vi "setVipBuildNumber.vi"() -> ()   [LabVIEW 2015]
uses:
  <vilib>/JKI/VIPM API/command-line/support/VI Package Build Spec Data Cluster_vipm_api.ctl
  <vilib>/JKI/VIPM API/command-line/support/Version Info Cluster_vipm_api.ctl
  <vilib>/Utility/error.llb/DialogType.ctl
  <vilib>/JKI/VIPM API/VIPM API_vipm_api.lvlib
  <vilib>/Wiresmith Technology/G CLI/CLI Class/CLI.lvclass
panel:
  out "Next build number":u32
  out "error out":errorcluster
  out "VI Package Build Spec Data":T1
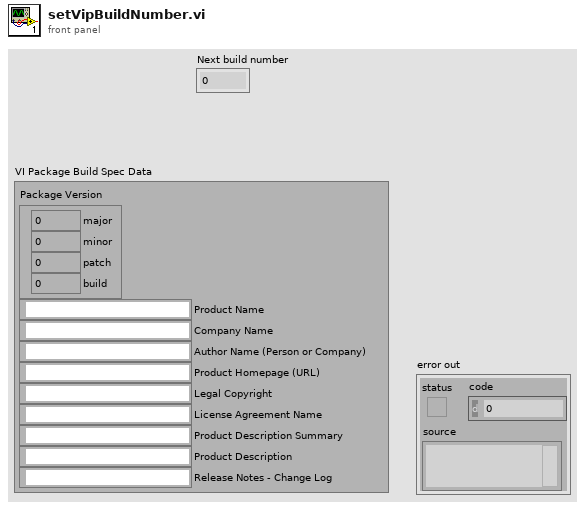
[diagram p1: front panel]
types:
  T1 = typedef "VIPM API_vipm_api.lvlib/VI Package Build Spec Data Cluster_vipm_api.ctl" = cluster{"Package Version":T2, "Product Name":string, "Company Name":string, "Author Name (Person or Company)":string, "Product Homepage (URL)":string, "Legal Copyright":string, "License Agreement Name":string, "Product Description Summary":string, "Product Description":string, "Release Notes - Change Log":string}
  T2 = typedef "VIPM API_vipm_api.lvlib/Version Info Cluster_vipm_api.ctl" = cluster{"major":u32, "minor":u32, "patch":u32, "build":u32}
  T3 = typedef "VIPM API_vipm_api.lvlib/Repository Contents Cluster_vipm_api.ctl" = cluster{"Package Name":string, "Version":string, "Display Name":string, "Release Date":string, "Deprecated":bool}
  T4 = typedef "DialogType.ctl" = u16
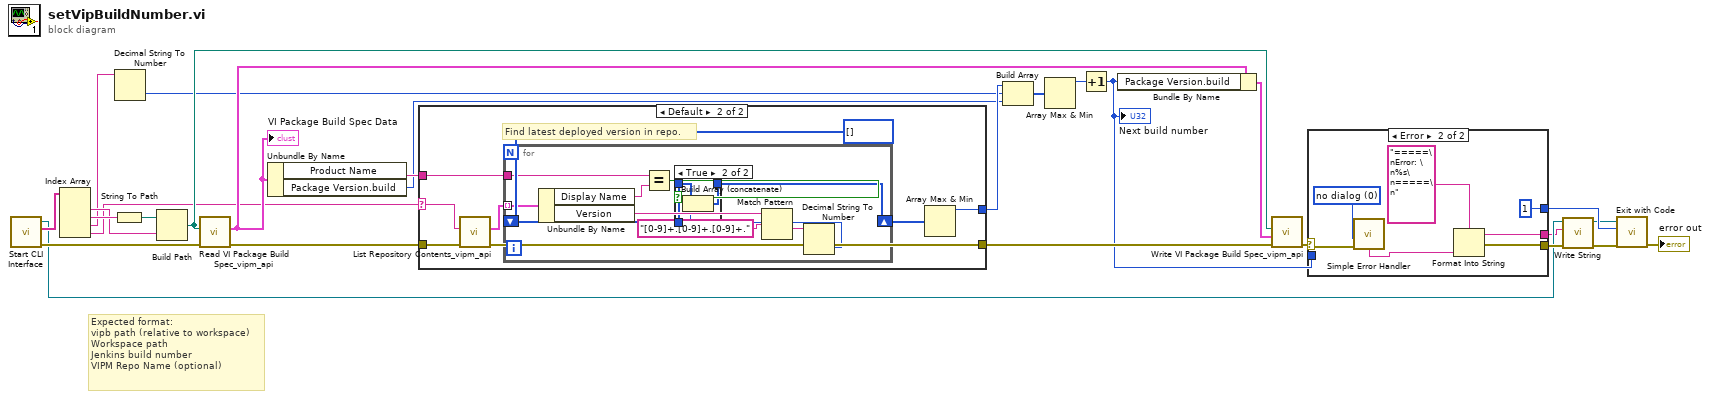
[diagram p0: block diagram]
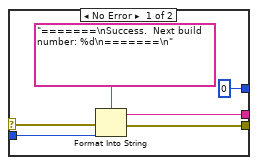
[diagram p2: hidden frame]
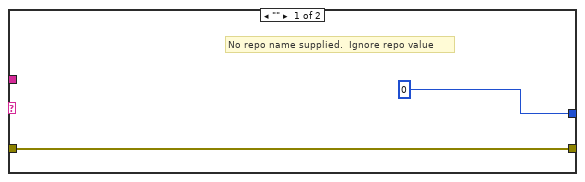
[diagram p3: hidden frame]
diagram:
  # "Expected format:\nvipb path (relative to workspace)\nWorkspace path\nJenkins build number\nVIPM Repo Name (optional)"
  n1 = call <vilib>:"Start CLI Interface.vi"() -> ("error out"=w18:errorcluster, "Custom Parameters"=w16:string[], "CLI out"=w3:refnum<class "CLI.lvclass">)  [unwired: 8 in, 1 out]
  n2 = Index Array(array=w16) -> (element #1=w13:string, element #2=w15:string, element #3=w12:string, element #4=w10:string)  [unwired: 4 in]
  n3 = String To Path(string=w15) -> (path=w14:path)
  n4 = Decimal String To Number(string=w12) -> (number=w11:i32)  [unwired: 2 in, 1 out]
  n5 = Build Path(base path=w14, name or relative path=w13) -> (appended path=w17:path)
  n6 = call <vilib>:"Read VI Package Build Spec_vipm_api.vi"("error in (no error)"=w18, "Path to VIPB File"=w17) -> ("error out"=w23:errorcluster, "VI Package Build Spec Data"=w22:T1)  [unwired: 8 in]
  "VI Package Build Spec Data" <- w22
  n7 = Unbundle By Name(w22) -> ("Product Name"=w21:string, "Package Version.build"=w20:u32)
  n8 = case shown="Default" w10 {
    selector: w10 -> [_ w33]
    tunnel: [0 w31] -> w27
    tunnel: [w28 w36] -> w7
    tunnel: w23 -> [w28 w35]
    tunnel: w21 -> [_ w34]
    frame "" {
      # "No repo name supplied.  Ignore repo value"
    }
    frame Default {
      # "Find latest deployed version in repo."
      n9 = call <vilib>:"List Repository Contents_vipm_api.vi"("error in (no error)"=w35, "Repository Name"=w33) -> ("error out"=w36:errorcluster, "Repository Contents []"=w37:T3[])  [unwired: 7 in, 1 out]
      n10 = for {
        tunnel: w37 -> [w47] mode=indexing
        tunnel: w34 -> [w45]
        shift-right: [w38] -> w32
        shift-left: i32[] [] ("Array") -> [w39]
        n11 = Unbundle By Name(w47) -> ("Display Name"=w46:string, "Version"=w42:string)
        n12 = Equal?(x=w45, y=w46) -> (x = y?=w40:bool)
        n13 = Match Pattern(string=w42, regular expression="[0-9]+.[0-9]+.[0-9]+.") -> (after substring=w43:string)  [unwired: 1 in, 3 out]
        n14 = Decimal String To Number(string=w43) -> (number=w41:i32)  [unwired: 2 in, 1 out]
        n15 = case shown="True" w40 {
          tunnel: w39 -> [w48 w50]
          tunnel: w41 -> [_ w49]
          tunnel: [w48 w51] -> w38
          frame False {
          }
          frame True {
            n16 = Build Array (concatenate)(w50, w49) -> (w51:i32[])
          }
        }
      }
      n17 = Array Max & Min(array=w32) -> (max value=w31:i32)  [unwired: 3 out]
    }
  }
  n18 = Build Array(w27, w11, w20) -> (w26:u32[])
  n19 = Array Max & Min(array=w26) -> (max value=w25:u32)  [unwired: 3 out]
  n20 = Increment(x=w25) -> (x+1=w6:u32)
  "Next build number" <- w6
  n21 = Bundle By Name(cluster=w22, "Package Version.build"=w6) -> (w24:T1)
  n22 = call <vilib>:"Write VI Package Build Spec_vipm_api.vi"("error in (no error)"=w7, "VI Package Build Spec Data"=w24, "Path to VIPB File"=w17) -> ("error out"=w9:errorcluster)  [unwired: 8 in]
  n23 = case shown="Error" w9 {
    selector: w9 -> [w55 w61]
    tunnel: [0 ("Exit Code (0)") 1 ("Exit Code (0)")] -> w8
    tunnel: w6 -> [w54 _]
    tunnel: [w53 w63] -> w4
    tunnel: [w52 w62] -> w2
    frame No Error {
      n24 = Format Into String(format string="=======\nSuccess.  Next build number: %d\n=======\n", error in=w55, w54) -> (resulting string=w52:string, error out=w53:errorcluster)  [unwired: 1 in]
    }
    frame Error {
      w58 = T4 0 items=["no dialog", "OK message", "continue or stop message", "OK message + warnings", "continue/stop + warnings"] ("type of dialog (OK msg:1)")
      n25 = call <vilib>:"Simple Error Handler.vi"("type of dialog (OK msg:1)"=w58, "error in (no error)"=w61) -> ("message"=w59:string)  [unwired: 3 in, 4 out]
      n26 = Format Into String(format string="=====\nError: \n%s\n=====\n", w59) -> (resulting string=w62:string, error out=w63:errorcluster)  [unwired: 2 in]
    }
  }
  n27 = call <vilib>:"Write String.vi"("error in (no error)"=w4, "Text to Write"=w2, "CLI in"=w3) -> ("error out"=w5:errorcluster, "CLI out"=w1:refnum<class "CLI.lvclass">)  [unwired: 7 in]
  n28 = call <vilib>:"Exit with Code.vi"("error in (no error)"=w5, "Exit Code (0)"=w8, "CLI in"=w1) -> ("error out"=→"error out":errorcluster)  [unwired: 8 in]
